vi "macro_MatBuilder_Create.vi"   [LabVIEW 2019, in "Trajectory_Library.lvlib"]
uses:
  Trajectory_Library.lvlib
  DCMOTOR_TYPES_ENUM.ctl
types:
  T1 = typedef "Trajectory_Library.lvlib/DCMOTOR_TYPES_ENUM.ctl" = enum16{"CIM", "AndyMark 9015", "Andy Mark RS 775 125", "Bag", "BaneBots RS 550", "BaneBots RS 775", "Falcon 500", "Mini CIM", "NEO", "NEO 550", "Romi BuiltIn", "Vex 775 Pro"}
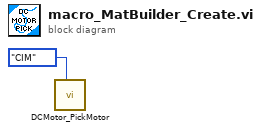
[diagram p0: block diagram]
diagram:
  n1 = call "DCMotor_PickMotor.vi"("DCMOTOR_TYPES"=DCMOTOR_TYPES_ENUM."CIM") -> ()  [unwired: 10 in, 1 out]
